vi "file_name_tracer.vi"(1 "input path string":string) -> (0 "file name":string)   [LabVIEW 2014]
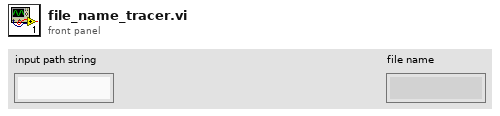
[diagram p1: front panel]
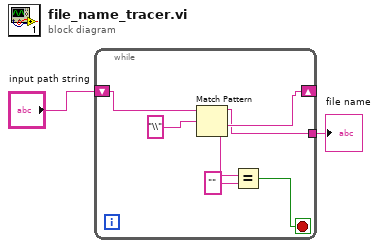
[diagram p0: block diagram]
diagram:
  n1 = while {
    shift-right: [w5] -> _
    shift-left: "input path string" -> [w4]
    tunnel: [w3] -> w1
    stop <- w8 stop-if-true
    n2 = Match Pattern(string=w4, regular expression="\\") -> (before substring=w3:string, match substring=w7:string, after substring=w5:string)  [unwired: 1 in, 1 out]
    n3 = Equal?(x=w7, y="") -> (x = y?=w8:bool)
  }
  "file name" <- w1
